vi "Subvi DO.vi"(2 "DO channel":refnum<k21>="Connector1/DIO0", 10 "Memory label":refnum<k21>="DO0 buffer") -> ()   [LabVIEW 2017]
uses:
  <vilib>/Platform/TimedLoop/XDataNode/timing_clust.ctl
  <vilib>/Platform/TimedLoop/XDataNode/nitl_modes.ctl
  <vilib>/Platform/TimedLoop/XDataNode/wakeup.ctl
  Control/GV DO delay.vi
  <vilib>/rvi/Emulation/niFpgaSctlEmulationGetInTimedLoop.vi
  <vilib>/rvi/Emulation/niFpgaEmulationReportErrorSimple.vi
  <vilib>/rvi/Emulation/niFpgaGetClockAttributes.vi
  <vilib>/rvi/Emulation/niFpgaCriticalErrorInLSC.vi
  Control/GV input buffer ready.vi
  <vilib>/rvi/DataTransferAndStorage/Container/Common/niFpgaContainerExecOnDevCompGetState.vi
  <vilib>/rvi/Emulation/niFpgaEmulationIsFPGAContextNoSignature.vi
  <vilib>/rvi/DataTransferAndStorage/Container/Common/niFpgaContainerGetUniqueNameForEmu.vi
  <vilib>/rvi/Emulation/niFpgaProcessEmulError.vi
  <vilib>/rvi/errors/nirviReportUnexpectedCaseInternalError (U32).vi
  <vilib>/rvi/Memory/Memory_Emulation/niFpgaMemoryEmulationCacheClearOnFirstRun.vi
  <vilib>/rvi/Memory/Memory_Emulation/nirvimemoryEmulationManagerCache_MakeExclusive.vi
  <vilib>/rvi/Memory/Memory_Emulation/niFpgaMemoryEmulationValidateCache.vi
  <vilib>/rvi/Memory/Memory_Emulation/nirvimemoryEmulationManagerCache_InsertValue.vi
  <vilib>/Utility/error.llb/Clear Errors.vi
  <vilib>/rvi/Memory/Memory_Emulation/nirvimemoryEmulationManagerCache_ReleaseExclusive.vi
  <vilib>/rvi/Memory/Memory_Emulation/nirvimemoryEmulationManagerCache_GetValue.vi
  <vilib>/rvi/Memory/Memory_Emulation/nirvimemoryEmulationManagerCache_SetValue.vi
  <vilib>/rvi/Emulation/niFpgaSctlEmulationResourceMgr.vi
  <vilib>/rvi/eio/common/nirviEmuTemplateMethod_errors.vi
  <vilib>/Platform/TimedLoop/XDataNode/XDataNode.xnode
  <vilib>/rvi/DataTransferAndStorage/Container/XNode/niFpgaContainer.xnode
  <vilib>/rvi/Memory/Memory_Emulation/niFpgaMemoryEmulationRefIn.vi
  <vilib>/eio/EIONode/EIONode.xnode
  <vilib>/Platform/TimedLoop/XDataNode/XDNodeRunTimeDep.lvlib
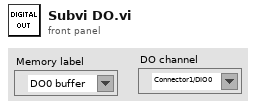
[diagram p1: front panel]
types:
  T1 = typedef "XDNodeRunTimeDep.lvlib/timing_clust.ctl" = cluster{"Expected End [f-1]":u64, "Actual End [f-1]":u64, "Finished Late? [f-1]":bool, "Expected End [i-1]":u64, "Actual End [i-1]":u64, "Finished Late? [i-1]":bool, "Expected Start [i]":u64, "Actual Start [i]":u64, "Expected Start [f]":u64, "Actual Start [f]":u64, "Source Name":string, "Structure Name":string, "Period":i64, "Deadline":i64, "Offset":i64, "Start":i64, "Priority":i32, "Timeout":i32, "Mode":T2, "Wakeup Reason":T3, "Error":errorcluster, "Source Type":string, "Secondary Source Type":string, "Global End Time":u64, "Global Start Time":u64, "Frame Duration":u64, "Iteration Duration":u64, "Assigned CPU":i32, "I/O Scan Engine Mode":u32}
  T2 = typedef "XDNodeRunTimeDep.lvlib/nitl_modes.ctl" = enum32{"No Change", "Process missed periods, maintain original phase", "Discard missed periods, maintain original phase", "Process missed periods, ignore original phase", "Discard missed periods, ignore original phase"}
  T3 = typedef "XDNodeRunTimeDep.lvlib/wakeup.ctl" = enum32{"Normal", "Aborted", "Asynchronous wakeup", "Timing source error", "Timed loop error", "Timeout"}
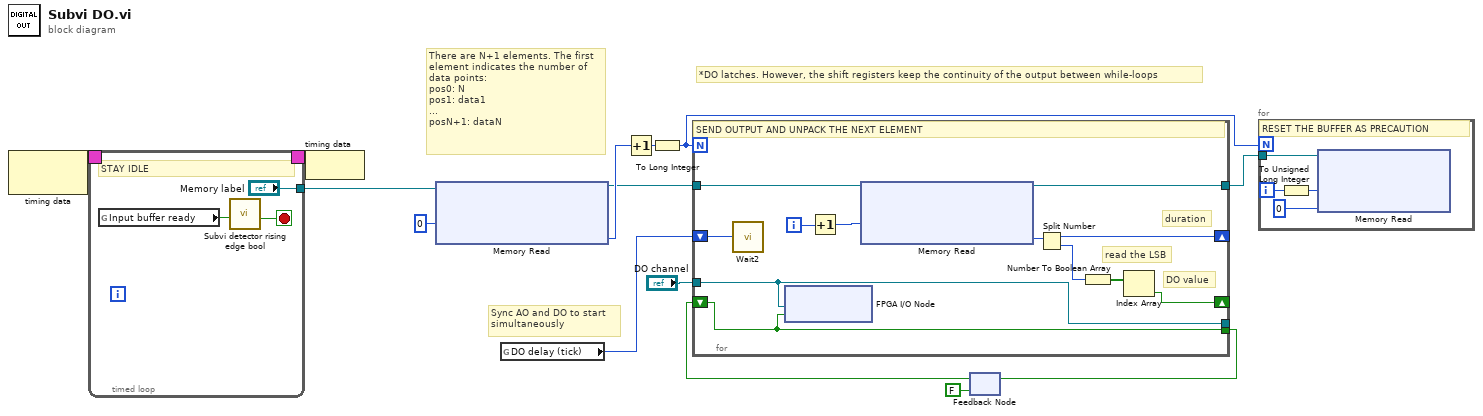
[diagram p0: block diagram]
diagram:
  # "There are N+1 elements. The first\nelement indicates the number of\ndata points:\npos0: N\npos1: data1\n...\nposN+1: dataN"
  # "*DO latches. However, the shift registers keep the continuity of the output between while-loops"
  # "Sync AO and DO to start\nsimultaneously"
  n1 = node-c288() -> (w5:T1)  [unwired: 1 in]
  n2 = timed-loop {
    timing: w5 -> [_]
    timing-out: [_] -> w4
    tunnel: ["Memory label"] -> w3
    stop <- w16 stop-if-true
    # "STAY IDLE"
    n3 = global read "GV input buffer ready.vi" "Input buffer ready"() -> (w17:bool)
    n4 = call "Subvi detector rising edge bool.vi"("Input"=w17) -> ("Output"=w16:bool)  [unwired: 10 in]
  }
  n5 = node-c288(w4) -> ()
  n6 = xnode ("Memory Read")("Address"=u32 0, "Memory In"=w3) -> ("Data"=w11:u32, "Memory Out"=w9:refnum<k21>)
  n7 = global read "GV DO delay.vi" "DO delay (tick)"() -> (w14:u16)
  n8 = Increment(x=w11) -> (x+1=w10:u32)
  n9 = To Long Integer(number=w10) -> (32bit integer=w8:i32)
  n10 = feedback #1(FALSE) -> (w6:bool)
  n11 = for {
    N: w8 -> [_]
    shift-right: [w26] -> _
    shift-left: w6 -> [w21]
    shift-right: [w28] -> _
    shift-left: w14 -> [w27]
    tunnel: [w25] -> w12
    tunnel: w9 -> [w24]
    tunnel: [w21] -> w1
    tunnel: "DO channel" -> [w20]
    tunnel: [w20] -> _
    i -> [w23]
    # "read the LSB"
    # "DO value"
    # "duration"
    # "SEND OUTPUT AND UNPACK THE NEXT ELEMENT"
    n12 = call "Wait2"("Count(Ticks)"=w27) -> ()  [unwired: 1 out]
    n13 = xnode "FPGA I/O Node"("I/O Item"=w21, "FPGA I/O In"=w20) -> ()  [unwired: 1 out]
    n14 = Increment(x=w23) -> (x+1=w22:i32)
    n15 = xnode ("Memory Read")("Address"=w22, "Memory In"=w24) -> ("Data"=w30:u32, "Memory Out"=w25:refnum<k21>)
    n16 = Split Number(x=w30) -> (hi(x)=w28:u16, lo(x)=w29:u16)
    n17 = Number To Boolean Array(number=w29) -> (Boolean array=w31:bool[])
    n18 = Index Array(array=w31) -> (element=w26:bool)  [unwired: 1 in]
  }
  n19 = feedback-in #1(w1) -> ()
  n20 = for {
    N: w8 -> [_]
    tunnel: w12 -> [w35]
    i -> [w34]
    # "RESET THE BUFFER AS PRECAUTION"
    n21 = To Unsigned Long Integer(number=w34) -> (unsigned 32bit integer=w32:u32)
    n22 = xnode ("Memory Read")("Address"=w32, "Data"=u32 0, "Memory In"=w35) -> ()  [unwired: 1 out]
  }
